vi "32路模拟量输入.vi"() -> ()   [LabVIEW 2010]
uses:
  全局量/全局_配置.vi
panel:
  in  "同步_1":i32
  in  "数组_反馈值":dbl[][](array[numeric])
  in  "第几个数据":i32
  in  "第几组数据":i32
  out "数组_AD幅值":sgl[](array[numeric])
  out "数组_DSP幅值":sgl[](array[numeric])
  in  "数组_设定值":dbl[][](array[numeric])
  in  "数组_选择":bool[](array[boolean])
  out "light_32":bool
  out "light_31":bool
  out "light_30":bool
  out "light_29":bool
  out "light_28":bool
  out "light_27":bool
  out "light_26":bool
  out "light_25":bool
  out "light_24":bool
  out "light_23":bool
  out "light_22":bool
  out "light_21":bool
  out "light_20":bool
  out "light_19":bool
  out "light_18":bool
  out "light_17":bool
  out "Analog_back":string[][](table) caption="表格"
  in  "A_32":bool
  in  "A_31":bool
  in  "A_30":bool
  in  "A_29":bool
  in  "A_28":bool
  in  "A_27":bool
  in  "A_26":bool
  in  "A_25":bool
  in  "A_24":bool
  in  "A_23":bool
  in  "A_22":bool
  in  "A_21":bool
  in  "A_20":bool
  in  "A_19":bool
  in  "A_18":bool
  in  "A_17":bool
  out "合格？":bool[][](array[boolean])
  out "测试结论":string
  out "light_16":bool
  out "light_15":bool
  out "light_14":bool
  out "light_13":bool
  out "light_12":bool
  out "light_11":bool
  out "light_10":bool
  out "light_9":bool
  out "light_8":bool
  out "light_7":bool
  out "light_6":bool
  out "light_5":bool
  out "light_4":bool
  out "light_3":bool
  out "light_2":bool
  out "light_1":bool
  out "退出？":bool
  in  "btn_反选":bool
  in  "btn_全选":bool
  in  "A_16":bool
  in  "A_15":bool
  in  "A_14":bool
  in  "A_13":bool
  in  "A_12":bool
  in  "A_11":bool
  in  "A_10":bool
  in  "A_9":bool
  in  "A_8":bool
  in  "A_7":bool
  in  "A_6":bool
  in  "A_5":bool
  in  "A_4":bool
  in  "A_3":bool
  in  "A_2":bool
  in  "A_1":bool
  in  "btn_取消":bool
  in  "btn_开始测试":bool
  in  "Analog_IN":string[][](table) caption="表格"
  out "Analog_WC":string[][](table) caption="表格"
  # "模拟量选择及输入值（V）"
  # "模拟量反馈值（V）"
  # "模拟量误差值（%）"
  # "测试结论："
  # "从0开始"
  # "从1开始,第0列没有使用"
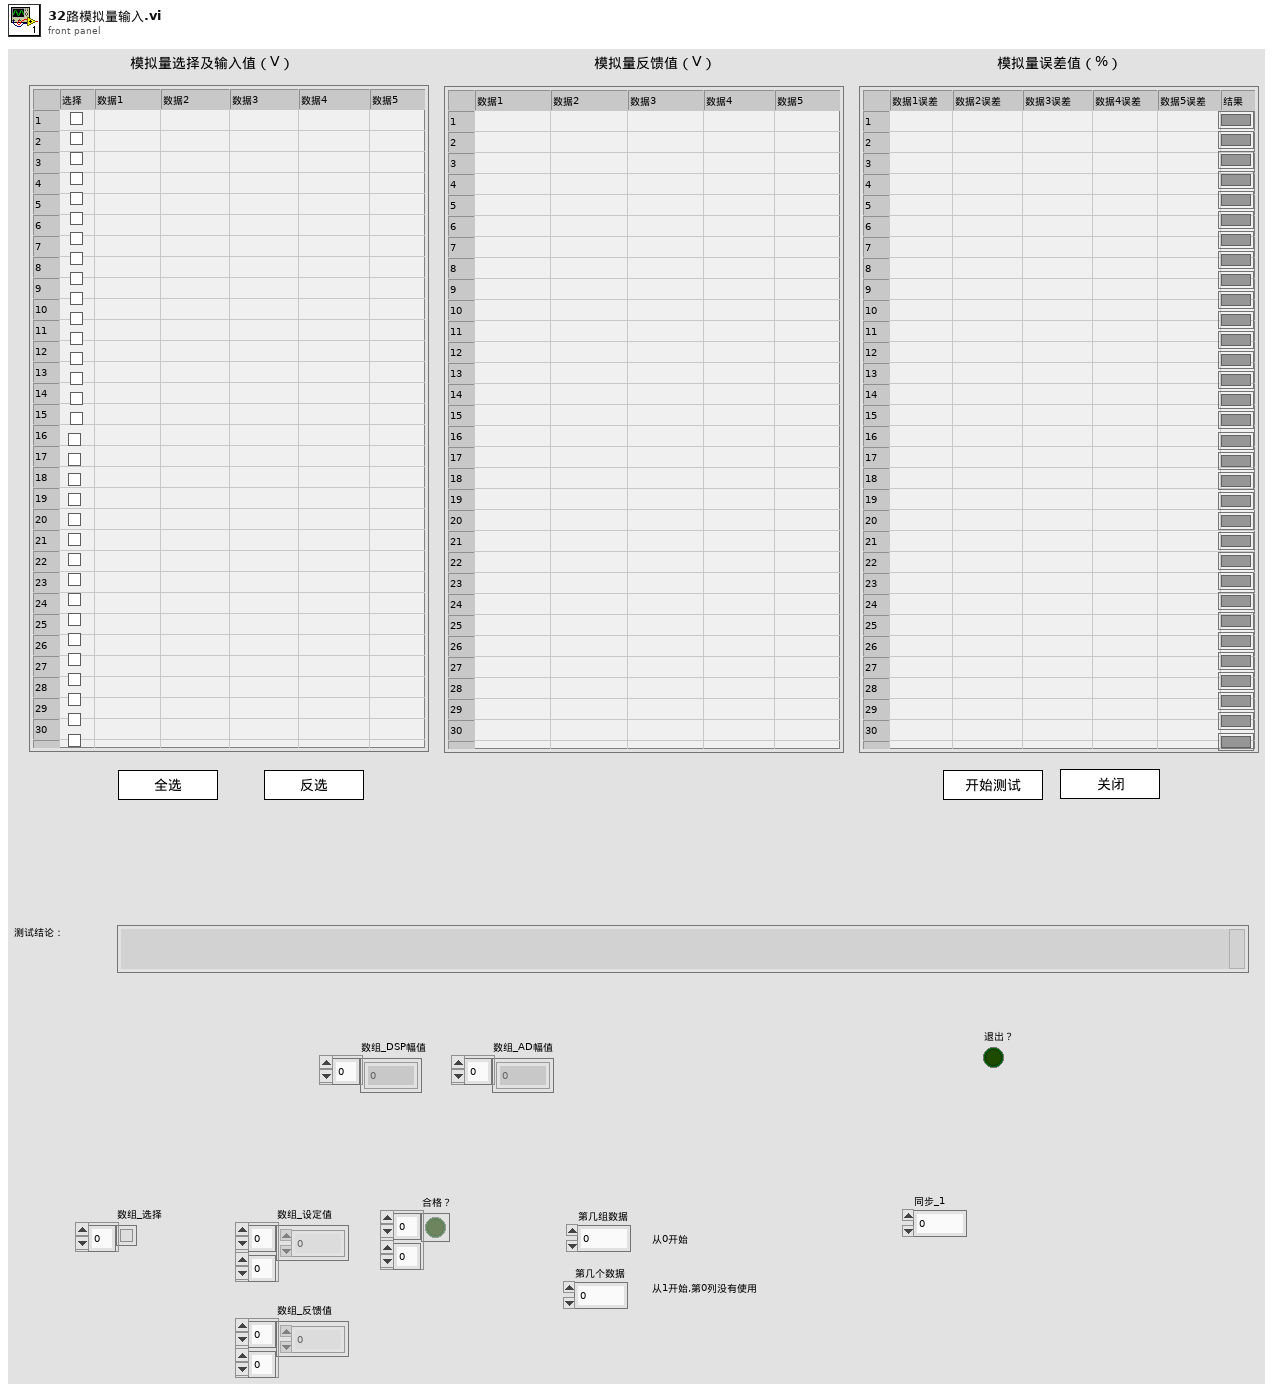
[diagram p1: front panel]
types:
  T1 = enum8{"Enabled", "Disabled", "Disabled and Grayed Out"}
  T2 = cluster{"数字量输入信号路数":u32, "数字量输出信号路数":u32, "DSP模拟量输入信号路数":u32, "DSP模拟量输入信号幅值":u32, "AD模拟量输入信号路数":u32, "AD模拟量输入信号幅值":u32, "RS232端口":u32, "RS232通信路数":u32, "RS232波特率":u32, "RS485端口":u32, "RS485通信路数":u32, "RS485波特率":u32, "CAN通信端口":string, "CAN波特率":u32, "以太网选择?":bool, "控制板IP":string, "以太网端口":u32}
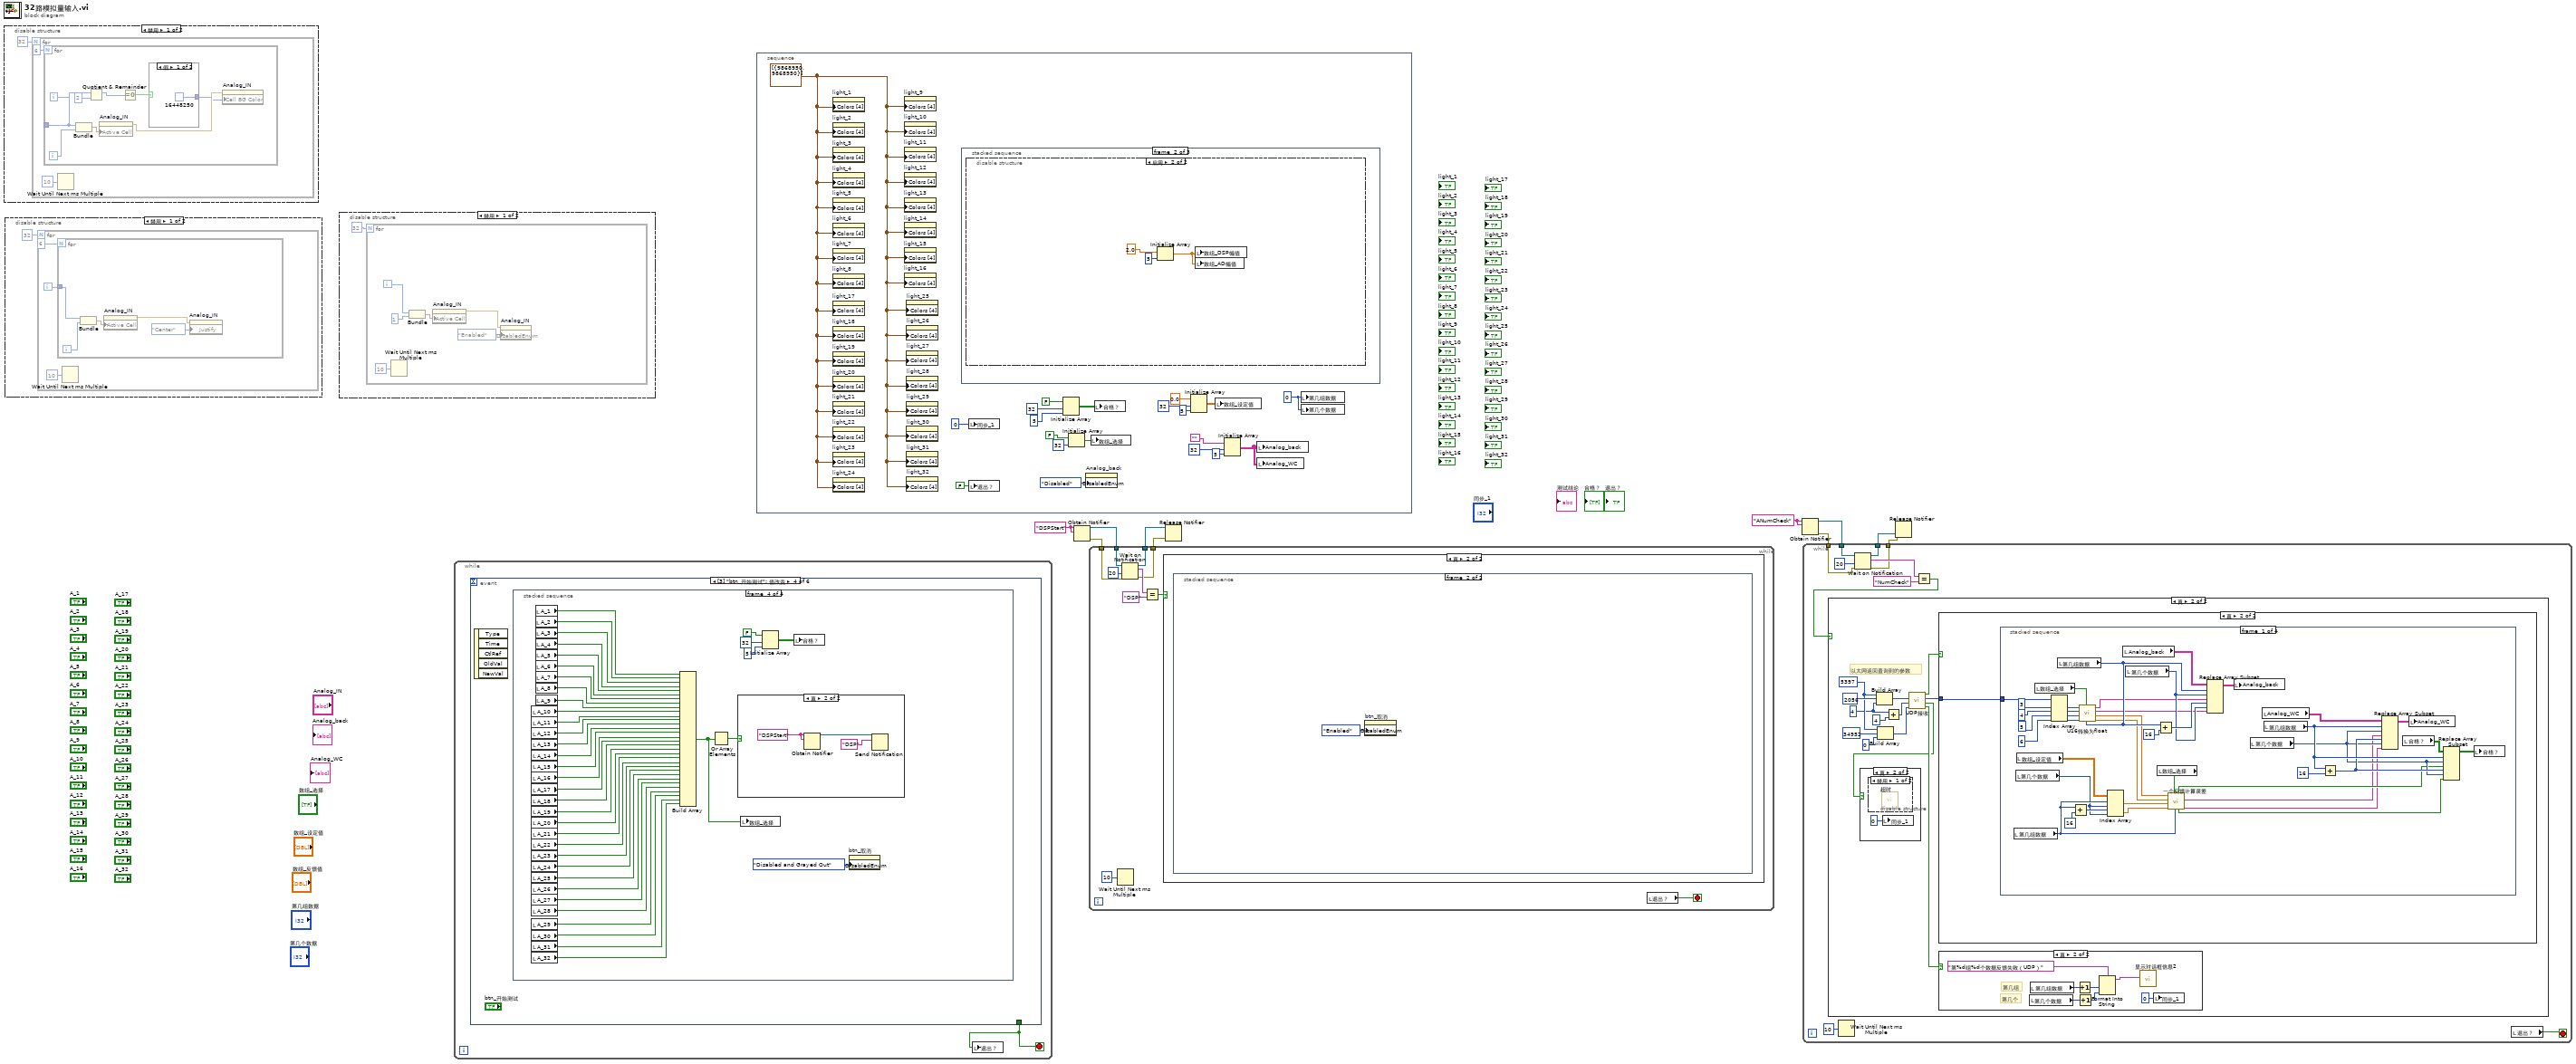
[diagram p0: block diagram]
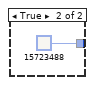
[diagram p2: hidden frame]
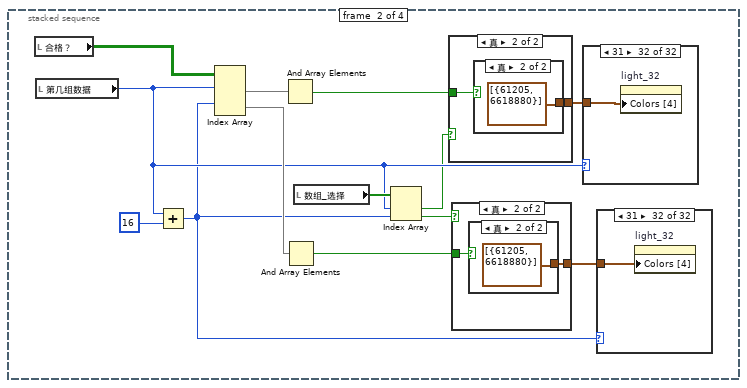
[diagram p9: hidden frame]
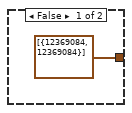
[diagram p10: hidden frame]
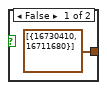
[diagram p11: hidden frame]
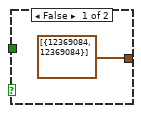
[diagram p12: hidden frame]
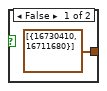
[diagram p13: hidden frame]
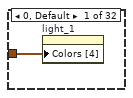
[diagram p14: hidden frame]
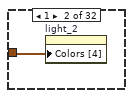
[diagram p15: hidden frame]
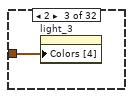
[diagram p16: hidden frame]
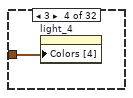
[diagram p17: hidden frame]
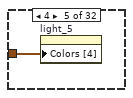
[diagram p18: hidden frame]
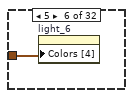
[diagram p19: hidden frame]
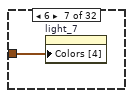
[diagram p20: hidden frame]
diagram:
  w5 = "ANumCheck" ("名称（未命名）")
  w8 = "DSPStart" ("名称（未命名）")
  n1 = disable-structure shown="禁用" {
    frame Disabled {
      n2 = for {
        N: 32 -> [_]
        i -> [w13]
        n3 = for {
          N: 6 -> [_]
          tunnel: w13 -> [w21]
          i -> [w15]
          n4 = Bundle(w21, w15) -> (w18:cluster{i32, i32})  [unwired: 1 in]
          n5 = Quotient & Remainder(x=w21, y=2) -> (x-y*floor(x/y)=w19:i32)  [unwired: 1 out]
          n6 = property on="Analog_IN" class="Tbl (严格)"("Active Cell"=w18) -> (error out=w17:errorcluster)  [unwired: 2 in, 1 out]
          n7 = Equal To 0?(x=w19) -> (x = 0?=w22:bool)
          n8 = case shown="假" w22 {
            tunnel: [u32 16448250 u32 15723488] -> w16
            frame False {
            }
            frame True {
            }
          }
          n9 = property on="Analog_IN" class="Tbl (严格)"(error in=w17, "Cell BG Color"=w16) -> ()  [unwired: 1 in, 2 out]
        }
        n10 = Wait Until Next ms Multiple(millisecond multiple=u32 10 ("毫秒倍数")) -> ()  [unwired: 1 out]
      }
    }
    frame Enabled {
    }
  }
  n11 = disable-structure shown="禁用" {
    frame Disabled {
      n12 = for {
        N: 32 -> [_]
        i -> [w26]
        n13 = for {
          N: 6 -> [_]
          tunnel: w26 -> [w29]
          i -> [w30]
          n14 = Bundle(w29, w30) -> (w33:cluster{i32, i32})  [unwired: 1 in]
          n15 = property on="Analog_IN" class="Tbl (严格)"("Active Cell"=w33) -> (error out=w31:errorcluster)  [unwired: 2 in, 1 out]
          n16 = property on="Analog_IN" class="Tbl (严格)"(error in=w31, "Justify"=enum16{"Left", "Center", "Right"}."Center" ("活动单元格:单元格对齐")) -> ()  [unwired: 1 in, 2 out]
        }
        n17 = Wait Until Next ms Multiple(millisecond multiple=u32 10 ("毫秒倍数")) -> ()  [unwired: 1 out]
      }
    }
    frame Enabled {
    }
  }
  n18 = disable-structure shown="禁用" {
    frame Disabled {
      n19 = for {
        N: 32 -> [_]
        i -> [w39]
        n20 = Wait Until Next ms Multiple(millisecond multiple=u32 10 ("毫秒倍数")) -> ()  [unwired: 1 out]
        n21 = Bundle(w39, 1) -> (w38:cluster{i32, i32})  [unwired: 1 in]
        n22 = property on="Analog_IN" class="Tbl (严格)"("Active Cell"=w38) -> (error out=w35:errorcluster)  [unwired: 2 in, 1 out]
        n23 = property on="Analog_IN" class="Tbl (严格)"(error in=w35, "DisabledEnum"=T1."Enabled" ("禁用")) -> ()  [unwired: 1 in, 2 out]
      }
    }
    frame Enabled {
    }
  }
  n24 = while {
    stop <- w41 stop-if-true
    n25 = event shown="[3] \"btn_开始测试\": 值改变" {
      selector: _ -> [_ _ _ _ _ _]
      dyn-events: _ -> [_ _ _ _ _ _]
      timeout: _ -> [_ _ _ _ _ _]
      tunnel: [_ TRUE TRUE _ _ _] -> w41
      event Timeout {
        n26 = event-data() -> ()  [unwired: 1 in, 2 out]
      }
      event Panel Close {
        n27 = event-data() -> ()  [unwired: 1 in, 3 out]
      }
      event "btn_取消": Value Change {
        n28 = event-data() -> ()  [unwired: 1 in, 5 out]
      }
      event "btn_开始测试": Value Change {
        n29 = event-data() -> ()  [unwired: 1 in, 5 out]
        n30 = stacked-sequence {
          frame #0 {
            w44 = 0 ("第几组数据")
            n31 = local read "Analog_IN"() -> (w51:string[][])
            n32 = Delete From Array(array=w51, length=1 ("长度"), index (col)=0 ("禁用的索引 (列)")) -> (array with subset deleted=w47:string[][])  [unwired: 1 in, 1 out]
            n33 = for {
              N: 32 -> [_]
              tunnel: w47 -> [w54] mode=indexing
              tunnel: [w53] -> w50 mode=indexing
              n34 = for {
                N: 5 -> [_]
                tunnel: w54 -> [w56] mode=indexing
                tunnel: [w55] -> w53 mode=indexing
                n35 = Fract/Exp String To Number(string=w56) -> (number=w55:dbl)  [unwired: 3 in, 1 out]
              }
            }
            n36 = local write "第几组数据"(w44) -> ()
            n37 = local write "第几个数据"(w44) -> ()
            n38 = local write "同步_1"(0 ("同步_2")) -> ()
            n39 = local write "数组_设定值"(w50) -> ()
          }
          frame #1 {
            n40 = local read "Analog_back"() -> (w59:string[][])
            n41 = local read "Analog_WC"() -> (w58:string[][])
            n42 = for {
              tunnel: w58 -> [w95] mode=indexing
              i -> [w94]
              n43 = for {
                tunnel: w95 -> [_] mode=indexing
                tunnel: w94 -> [w99]
                i -> [w98]
                n44 = local read "Analog_WC"() -> (w100:string[][])
                n45 = Replace Array Subset(array=w100, new element="", index (row)=w99, index (col)=w98) -> (w96:string[][])
                n46 = local write "Analog_WC"(w96) -> ()
              }
            }
            n47 = for {
              tunnel: w59 -> [w102] mode=indexing
              i -> [w101]
              n48 = for {
                tunnel: w102 -> [_] mode=indexing
                tunnel: w101 -> [w106]
                i -> [w105]
                n49 = local read "Analog_back"() -> (w107:string[][])
                n50 = Replace Array Subset(array=w107, new element="", index (row)=w106, index (col)=w105) -> (w103:string[][])
                n51 = local write "Analog_back"(w103) -> ()
              }
            }
            n52 = for {
              N: 32 -> [_]
              i -> [w61]
              n53 = case shown="31" w61 {
                tunnel: cluster{u32, u32}[] [{9868950, 9868950}] -> [w62 w63 w64 w65 w66 w67 w68 w69 w70 w71 w72 w73 w74 w75 w76 w77 w78 w79 w80 w81 w82 w83 w84 w85 w86 w87 w88 w89 w90 w91 w92 w93]
                frame 0, Default {
                  n54 = property on="light_1" class="Bool (严格)"("Colors [4]"=w62) -> ()  [unwired: 2 in, 2 out]
                }
                frame 1 {
                  n55 = property on="light_2" class="Bool (严格)"("Colors [4]"=w63) -> ()  [unwired: 2 in, 2 out]
                }
                frame 2 {
                  n56 = property on="light_3" class="Bool (严格)"("Colors [4]"=w64) -> ()  [unwired: 2 in, 2 out]
                }
                frame 3 {
                  n57 = property on="light_4" class="Bool (严格)"("Colors [4]"=w65) -> ()  [unwired: 2 in, 2 out]
                }
                frame 4 {
                  n58 = property on="light_5" class="Bool (严格)"("Colors [4]"=w66) -> ()  [unwired: 2 in, 2 out]
                }
                frame 5 {
                  n59 = property on="light_6" class="Bool (严格)"("Colors [4]"=w67) -> ()  [unwired: 2 in, 2 out]
                }
                frame 6 {
                  n60 = property on="light_7" class="Bool (严格)"("Colors [4]"=w68) -> ()  [unwired: 2 in, 2 out]
                }
                frame 7 {
                  n61 = property on="light_8" class="Bool (严格)"("Colors [4]"=w69) -> ()  [unwired: 2 in, 2 out]
                }
                frame 8 {
                  n62 = property on="light_9" class="Bool (严格)"("Colors [4]"=w70) -> ()  [unwired: 2 in, 2 out]
                }
                frame 9 {
                  n63 = property on="light_10" class="Bool (严格)"("Colors [4]"=w71) -> ()  [unwired: 2 in, 2 out]
                }
                frame 10 {
                  n64 = property on="light_11" class="Bool (严格)"("Colors [4]"=w72) -> ()  [unwired: 2 in, 2 out]
                }
                frame 11 {
                  n65 = property on="light_12" class="Bool (严格)"("Colors [4]"=w73) -> ()  [unwired: 2 in, 2 out]
                }
                frame 12 {
                  n66 = property on="light_13" class="Bool (严格)"("Colors [4]"=w74) -> ()  [unwired: 2 in, 2 out]
                }
                frame 13 {
                  n67 = property on="light_14" class="Bool (严格)"("Colors [4]"=w75) -> ()  [unwired: 2 in, 2 out]
                }
                frame 14 {
                  n68 = property on="light_15" class="Bool (严格)"("Colors [4]"=w76) -> ()  [unwired: 2 in, 2 out]
                }
                frame 15 {
                  n69 = property on="light_16" class="Bool (严格)"("Colors [4]"=w77) -> ()  [unwired: 2 in, 2 out]
                }
                frame 16 {
                  n70 = property on="light_17" class="Bool (严格)"("Colors [4]"=w78) -> ()  [unwired: 2 in, 2 out]
                }
                frame 17 {
                  n71 = property on="light_18" class="Bool (严格)"("Colors [4]"=w79) -> ()  [unwired: 2 in, 2 out]
                }
                frame 18 {
                  n72 = property on="light_19" class="Bool (严格)"("Colors [4]"=w80) -> ()  [unwired: 2 in, 2 out]
                }
                frame 19 {
                  n73 = property on="light_20" class="Bool (严格)"("Colors [4]"=w81) -> ()  [unwired: 2 in, 2 out]
                }
                frame 20 {
                  n74 = property on="light_21" class="Bool (严格)"("Colors [4]"=w82) -> ()  [unwired: 2 in, 2 out]
                }
                frame 21 {
                  n75 = property on="light_22" class="Bool (严格)"("Colors [4]"=w83) -> ()  [unwired: 2 in, 2 out]
                }
                frame 22 {
                  n76 = property on="light_23" class="Bool (严格)"("Colors [4]"=w84) -> ()  [unwired: 2 in, 2 out]
                }
                frame 23 {
                  n77 = property on="light_24" class="Bool (严格)"("Colors [4]"=w85) -> ()  [unwired: 2 in, 2 out]
                }
                frame 24 {
                  n78 = property on="light_25" class="Bool (严格)"("Colors [4]"=w86) -> ()  [unwired: 2 in, 2 out]
                }
                frame 25 {
                  n79 = property on="light_26" class="Bool (严格)"("Colors [4]"=w87) -> ()  [unwired: 2 in, 2 out]
                }
                frame 26 {
                  n80 = property on="light_27" class="Bool (严格)"("Colors [4]"=w88) -> ()  [unwired: 2 in, 2 out]
                }
                frame 27 {
                  n81 = property on="light_28" class="Bool (严格)"("Colors [4]"=w89) -> ()  [unwired: 2 in, 2 out]
                }
                frame 28 {
                  n82 = property on="light_29" class="Bool (严格)"("Colors [4]"=w90) -> ()  [unwired: 2 in, 2 out]
                }
                frame 29 {
                  n83 = property on="light_30" class="Bool (严格)"("Colors [4]"=w91) -> ()  [unwired: 2 in, 2 out]
                }
                frame 30 {
                  n84 = property on="light_31" class="Bool (严格)"("Colors [4]"=w92) -> ()  [unwired: 2 in, 2 out]
                }
                frame 31 {
                  n85 = property on="light_32" class="Bool (严格)"("Colors [4]"=w93) -> ()  [unwired: 2 in, 2 out]
                }
              }
            }
          }
          frame #2 {
            n86 = for {
              N: 32 -> [_]
              i -> [w110]
              n87 = disable-structure shown="禁用" {
                frame Disabled {
                  n88 = Wait Until Next ms Multiple(millisecond multiple=u32 10 ("毫秒倍数")) -> ()  [unwired: 1 out]
                }
                frame Enabled {
                }
              }
              n89 = for {
                N: 6 -> [_]
                tunnel: w110 -> [w118]
                i -> [w115]
                n90 = Bundle(w118, w115) -> (w114:cluster{i32, i32})  [unwired: 1 in]
                n91 = Quotient & Remainder(x=w118, y=2) -> (x-y*floor(x/y)=w116:i32)  [unwired: 1 out]
                n92 = property on="Analog_WC" class="Tbl (严格)"("Active Cell"=w114) -> (error out=w113:errorcluster)  [unwired: 2 in, 1 out]
                n93 = Equal To 0?(x=w116) -> (x = 0?=w119:bool)
                n94 = case shown="假" w119 {
                  tunnel: [u32 16448250 u32 15723488] -> w112
                  frame False {
                  }
                  frame True {
                  }
                }
                n95 = property on="Analog_WC" class="Tbl (严格)"(error in=w113, "Cell BG Color"=w112) -> ()  [unwired: 1 in, 2 out]
              }
            }
          }
          frame #3 {
            n96 = local read "A_10"() -> (w151:bool)
            n97 = local read "A_11"() -> (w150:bool)
            n98 = local read "A_12"() -> (w149:bool)
            n99 = local read "A_13"() -> (w148:bool)
            n100 = local read "A_14"() -> (w147:bool)
            n101 = local read "A_15"() -> (w146:bool)
            n102 = local read "A_16"() -> (w145:bool)
            n103 = local read "A_17"() -> (w144:bool)
            n104 = local read "A_18"() -> (w143:bool)
            n105 = local read "A_19"() -> (w142:bool)
            n106 = local read "A_20"() -> (w141:bool)
            n107 = local read "A_21"() -> (w140:bool)
            n108 = local read "A_22"() -> (w139:bool)
            n109 = local read "A_23"() -> (w138:bool)
            n110 = local read "A_24"() -> (w137:bool)
            n111 = local read "A_25"() -> (w136:bool)
            n112 = local read "A_26"() -> (w135:bool)
            n113 = local read "A_27"() -> (w134:bool)
            n114 = local read "A_28"() -> (w133:bool)
            n115 = local read "A_29"() -> (w132:bool)
            n116 = local read "A_30"() -> (w131:bool)
            n117 = local read "A_31"() -> (w130:bool)
            n118 = local read "A_32"() -> (w129:bool)
            n119 = local read "A_1"() -> (w160:bool)
            n120 = local read "A_2"() -> (w159:bool)
            n121 = local read "A_3"() -> (w158:bool)
            n122 = local read "A_4"() -> (w157:bool)
            n123 = local read "A_5"() -> (w156:bool)
            n124 = local read "A_6"() -> (w155:bool)
            n125 = local read "A_7"() -> (w154:bool)
            n126 = local read "A_8"() -> (w153:bool)
            n127 = local read "A_9"() -> (w152:bool)
            n128 = Build Array(w160, w159, w158, w157, w156, w155, w154, w153, w152, w151, w150, w149, w148, w147, w146, w145, w144, w143, w142, w141, w140, w139, w138, w137, w136, w135, w134, w133, w132, w131, w130, w129) -> (w123:bool[])
            n129 = Or Array Elements(Boolean array=w123) -> (logical OR=w128:bool)
            n130 = case shown="真" w128 {
              frame False {
                n131 = call "显示对话框信息"() -> ()  [unwired: 10 in, 2 out]
              }
              frame True {
                w162 = "DSPStart" ("名称（未命名）")
                n132 = Obtain Notifier(name (unnamed)=w162, notification data type=w162) -> (notifier out=w161:refnum<notifier>)  [unwired: 2 in, 2 out]
                n133 = Send Notification(notification="DSP" ("通知"), notifier=w161) -> ()  [unwired: 1 in, 2 out]
              }
            }
            n134 = local write "数组_选择"(w123) -> ()
            n135 = Initialize Array(FALSE, 32 ("维数大小"), 5 ("维数大小")) -> (w124:bool[][])
            n136 = local write "合格？"(w124) -> ()
            n137 = property on="btn_取消" class="Bool"("DisabledEnum"=T1."Disabled and Grayed Out" ("禁用")) -> ()  [unwired: 2 in, 2 out]
          }
        }
      }
      event "btn_全选": Value Change {
        w164 = TRUE ("单选_AD_1")
        n138 = event-data() -> ()  [unwired: 1 in, 5 out]
        n139 = local write "A_1"(w164) -> ()
        n140 = local write "A_2"(w164) -> ()
        n141 = local write "A_3"(w164) -> ()
        n142 = local write "A_4"(w164) -> ()
        n143 = local write "A_5"(w164) -> ()
        n144 = local write "A_6"(w164) -> ()
        n145 = local write "A_7"(w164) -> ()
        n146 = local write "A_8"(w164) -> ()
        n147 = local write "A_9"(w164) -> ()
        n148 = local write "A_10"(w164) -> ()
        n149 = local write "A_11"(w164) -> ()
        n150 = local write "A_12"(w164) -> ()
        n151 = local write "A_13"(w164) -> ()
        n152 = local write "A_14"(w164) -> ()
        n153 = local write "A_15"(w164) -> ()
        n154 = local write "A_16"(w164) -> ()
        n155 = local write "A_17"(w164) -> ()
        n156 = local write "A_18"(w164) -> ()
        n157 = local write "A_19"(w164) -> ()
        n158 = local write "A_20"(w164) -> ()
        n159 = local write "A_21"(w164) -> ()
        n160 = local write "A_22"(w164) -> ()
        n161 = local write "A_23"(w164) -> ()
        n162 = local write "A_24"(w164) -> ()
        n163 = local write "A_25"(w164) -> ()
        n164 = local write "A_26"(w164) -> ()
        n165 = local write "A_27"(w164) -> ()
        n166 = local write "A_28"(w164) -> ()
        n167 = local write "A_29"(w164) -> ()
        n168 = local write "A_30"(w164) -> ()
        n169 = local write "A_31"(w164) -> ()
        n170 = local write "A_32"(w164) -> ()
      }
      event "btn_反选": Value Change {
        n171 = event-data() -> ()  [unwired: 1 in, 5 out]
        n172 = local read "A_17"() -> (w196:bool)
        n173 = local read "A_18"() -> (w194:bool)
        n174 = local read "A_19"() -> (w192:bool)
        n175 = local read "A_20"() -> (w190:bool)
        n176 = local read "A_21"() -> (w188:bool)
        n177 = local read "A_22"() -> (w186:bool)
        n178 = local read "A_23"() -> (w184:bool)
        n179 = local read "A_24"() -> (w182:bool)
        n180 = local read "A_25"() -> (w180:bool)
        n181 = local read "A_26"() -> (w178:bool)
        n182 = local read "A_27"() -> (w176:bool)
        n183 = local read "A_28"() -> (w174:bool)
        n184 = local read "A_29"() -> (w172:bool)
        n185 = local read "A_30"() -> (w170:bool)
        n186 = local read "A_31"() -> (w168:bool)
        n187 = local read "A_32"() -> (w166:bool)
        n188 = local read "A_1"() -> (w228:bool)
        n189 = local read "A_2"() -> (w226:bool)
        n190 = local read "A_3"() -> (w225:bool)
        n191 = local read "A_4"() -> (w224:bool)
        n192 = local read "A_5"() -> (w223:bool)
        n193 = local read "A_6"() -> (w222:bool)
        n194 = local read "A_7"() -> (w221:bool)
        n195 = local read "A_8"() -> (w220:bool)
        n196 = local read "A_9"() -> (w219:bool)
        n197 = local read "A_10"() -> (w218:bool)
        n198 = local read "A_11"() -> (w217:bool)
        n199 = local read "A_12"() -> (w216:bool)
        n200 = local read "A_13"() -> (w215:bool)
        n201 = local read "A_14"() -> (w214:bool)
        n202 = local read "A_15"() -> (w213:bool)
        n203 = local read "A_16"() -> (w212:bool)
        n204 = Not(x=w228) -> (.not. x?=w227:bool)
        n205 = Not(x=w226) -> (.not. x?=w197:bool)
        n206 = Not(x=w225) -> (.not. x?=w198:bool)
        n207 = Not(x=w224) -> (.not. x?=w199:bool)
        n208 = Not(x=w223) -> (.not. x?=w200:bool)
        n209 = Not(x=w222) -> (.not. x?=w201:bool)
        n210 = Not(x=w221) -> (.not. x?=w202:bool)
        n211 = Not(x=w220) -> (.not. x?=w203:bool)
        n212 = Not(x=w219) -> (.not. x?=w204:bool)
        n213 = Not(x=w218) -> (.not. x?=w205:bool)
        n214 = Not(x=w217) -> (.not. x?=w206:bool)
        n215 = Not(x=w216) -> (.not. x?=w207:bool)
        n216 = Not(x=w215) -> (.not. x?=w208:bool)
        n217 = Not(x=w214) -> (.not. x?=w209:bool)
        n218 = Not(x=w213) -> (.not. x?=w210:bool)
        n219 = Not(x=w212) -> (.not. x?=w211:bool)
        n220 = Not(x=w196) -> (.not. x?=w195:bool)
        n221 = Not(x=w194) -> (.not. x?=w193:bool)
        n222 = Not(x=w192) -> (.not. x?=w191:bool)
        n223 = Not(x=w190) -> (.not. x?=w189:bool)
        n224 = Not(x=w188) -> (.not. x?=w187:bool)
        n225 = Not(x=w186) -> (.not. x?=w185:bool)
        n226 = Not(x=w184) -> (.not. x?=w183:bool)
        n227 = Not(x=w182) -> (.not. x?=w181:bool)
        n228 = Not(x=w180) -> (.not. x?=w179:bool)
        n229 = Not(x=w178) -> (.not. x?=w177:bool)
        n230 = Not(x=w176) -> (.not. x?=w175:bool)
        n231 = Not(x=w174) -> (.not. x?=w173:bool)
        n232 = Not(x=w172) -> (.not. x?=w171:bool)
        n233 = Not(x=w170) -> (.not. x?=w169:bool)
        n234 = Not(x=w168) -> (.not. x?=w167:bool)
        n235 = Not(x=w166) -> (.not. x?=w165:bool)
        n236 = local write "A_1"(w227) -> ()
        n237 = local write "A_2"(w197) -> ()
        n238 = local write "A_3"(w198) -> ()
        n239 = local write "A_4"(w199) -> ()
        n240 = local write "A_5"(w200) -> ()
        n241 = local write "A_6"(w201) -> ()
        n242 = local write "A_7"(w202) -> ()
        n243 = local write "A_8"(w203) -> ()
        n244 = local write "A_9"(w204) -> ()
        n245 = local write "A_10"(w205) -> ()
        n246 = local write "A_11"(w206) -> ()
        n247 = local write "A_12"(w207) -> ()
        n248 = local write "A_13"(w208) -> ()
        n249 = local write "A_14"(w209) -> ()
        n250 = local write "A_15"(w210) -> ()
        n251 = local write "A_16"(w211) -> ()
        n252 = local write "A_17"(w195) -> ()
        n253 = local write "A_18"(w193) -> ()
        n254 = local write "A_19"(w191) -> ()
        n255 = local write "A_20"(w189) -> ()
        n256 = local write "A_21"(w187) -> ()
        n257 = local write "A_22"(w185) -> ()
        n258 = local write "A_23"(w183) -> ()
        n259 = local write "A_24"(w181) -> ()
        n260 = local write "A_25"(w179) -> ()
        n261 = local write "A_26"(w177) -> ()
        n262 = local write "A_27"(w175) -> ()
        n263 = local write "A_28"(w173) -> ()
        n264 = local write "A_29"(w171) -> ()
        n265 = local write "A_30"(w169) -> ()
        n266 = local write "A_31"(w167) -> ()
        n267 = local write "A_32"(w165) -> ()
      }
    }
    n268 = local write "退出？"(w41) -> ()
  }
  n269 = stacked-sequence {
    frame #0 {
      w229 = 0 ("第几组数据")
      w244 = cluster{u32, u32}[] [{9868950, 9868950}]
      n270 = property on="light_1" class="Bool (严格)"("Colors [4]"=w244) -> ()  [unwired: 2 in, 2 out]
      n271 = property on="light_2" class="Bool (严格)"("Colors [4]"=w244) -> ()  [unwired: 2 in, 2 out]
      n272 = property on="light_3" class="Bool (严格)"("Colors [4]"=w244) -> ()  [unwired: 2 in, 2 out]
      n273 = property on="light_4" class="Bool (严格)"("Colors [4]"=w244) -> ()  [unwired: 2 in, 2 out]
      n274 = property on="light_5" class="Bool (严格)"("Colors [4]"=w244) -> ()  [unwired: 2 in, 2 out]
      n275 = property on="light_6" class="Bool (严格)"("Colors [4]"=w244) -> ()  [unwired: 2 in, 2 out]
      n276 = property on="light_7" class="Bool (严格)"("Colors [4]"=w244) -> ()  [unwired: 2 in, 2 out]
      n277 = property on="light_8" class="Bool (严格)"("Colors [4]"=w244) -> ()  [unwired: 2 in, 2 out]
      n278 = property on="light_17" class="Bool (严格)"("Colors [4]"=w244) -> ()  [unwired: 2 in, 2 out]
      n279 = property on="light_18" class="Bool (严格)"("Colors [4]"=w244) -> ()  [unwired: 2 in, 2 out]
      n280 = property on="light_19" class="Bool (严格)"("Colors [4]"=w244) -> ()  [unwired: 2 in, 2 out]
      n281 = property on="light_20" class="Bool (严格)"("Colors [4]"=w244) -> ()  [unwired: 2 in, 2 out]
      n282 = property on="light_21" class="Bool (严格)"("Colors [4]"=w244) -> ()  [unwired: 2 in, 2 out]
      n283 = property on="light_22" class="Bool (严格)"("Colors [4]"=w244) -> ()  [unwired: 2 in, 2 out]
      n284 = property on="light_23" class="Bool (严格)"("Colors [4]"=w244) -> ()  [unwired: 2 in, 2 out]
      n285 = property on="light_24" class="Bool (严格)"("Colors [4]"=w244) -> ()  [unwired: 2 in, 2 out]
      n286 = property on="light_9" class="Bool (严格)"("Colors [4]"=w244) -> ()  [unwired: 2 in, 2 out]
      n287 = property on="light_10" class="Bool (严格)"("Colors [4]"=w244) -> ()  [unwired: 2 in, 2 out]
      n288 = property on="light_11" class="Bool (严格)"("Colors [4]"=w244) -> ()  [unwired: 2 in, 2 out]
      n289 = property on="light_12" class="Bool (严格)"("Colors [4]"=w244) -> ()  [unwired: 2 in, 2 out]
      n290 = property on="light_13" class="Bool (严格)"("Colors [4]"=w244) -> ()  [unwired: 2 in, 2 out]
      n291 = property on="light_14" class="Bool (严格)"("Colors [4]"=w244) -> ()  [unwired: 2 in, 2 out]
      n292 = property on="light_15" class="Bool (严格)"("Colors [4]"=w244) -> ()  [unwired: 2 in, 2 out]
      n293 = property on="light_16" class="Bool (严格)"("Colors [4]"=w244) -> ()  [unwired: 2 in, 2 out]
      n294 = property on="light_25" class="Bool (严格)"("Colors [4]"=w244) -> ()  [unwired: 2 in, 2 out]
      n295 = property on="light_26" class="Bool (严格)"("Colors [4]"=w244) -> ()  [unwired: 2 in, 2 out]
      n296 = property on="light_27" class="Bool (严格)"("Colors [4]"=w244) -> ()  [unwired: 2 in, 2 out]
      n297 = property on="light_28" class="Bool (严格)"("Colors [4]"=w244) -> ()  [unwired: 2 in, 2 out]
      n298 = property on="light_29" class="Bool (严格)"("Colors [4]"=w244) -> ()  [unwired: 2 in, 2 out]
      n299 = property on="light_30" class="Bool (严格)"("Colors [4]"=w244) -> ()  [unwired: 2 in, 2 out]
      n300 = property on="light_31" class="Bool (严格)"("Colors [4]"=w244) -> ()  [unwired: 2 in, 2 out]
      n301 = property on="light_32" class="Bool (严格)"("Colors [4]"=w244) -> ()  [unwired: 2 in, 2 out]
      n302 = stacked-sequence {
        frame #0 {
          n303 = Initialize Array("", 32 ("维数大小"), 6 ("维数大小")) -> (w249:string[][])
          n304 = local write "Analog_IN"(w249) -> ()
        }
        frame #1 {
          n305 = disable-structure shown="启用" {
            frame Disabled {
              n306 = global read "全局_配置.vi" "BoardConfig"() -> (w257:T2)
              n307 = Unbundle By Name(w257) -> ("DSP模拟量输入信号幅值"=w256:u32, "AD模拟量输入信号幅值"=w255:u32)
              n308 = case shown="2" w255 {
                tunnel: [sgl 3.0 sgl 5.0 sgl 12.0] -> w253
                frame 0, Default {
                }
                frame 1 {
                }
                frame 2 {
                }
              }
              n309 = case shown="0, 默认" w256 {
                tunnel: [sgl 3.0 sgl 5.0 sgl 12.0] -> w254
                frame 0, Default {
                }
                frame 1 {
                }
                frame 2 {
                }
              }
              n310 = for {
                N: 5 -> [_]
                tunnel: w254 -> [w279]
                tunnel: w253 -> [w270]
                tunnel: [w268] -> w259 mode=indexing
                tunnel: [w267] -> w258 mode=indexing
                i -> [w282]
                n311 = Multiply(x=sgl 2.0, y=w279) -> (x*y=w277:sgl)
                n312 = Multiply(x=sgl 2.0, y=w270) -> (x*y=w274:sgl)
                n313 = case shown="4" w282 {
                  tunnel: [sgl 0.05 sgl 0.5 sgl 0.75 sgl 0.95 sgl 0.25] -> w269
                  frame 0, Default {
                  }
                  frame 2 {
                  }
                  frame 3 {
                  }
                  frame 4 {
                  }
                  frame 1 {
                  }
                }
                n314 = Multiply(x=w279, y=sgl -1.0) -> (x*y=w280:sgl)
                n315 = Multiply(x=w270, y=sgl -1.0) -> (x*y=w272:sgl)
                n316 = Multiply(x=w269, y=w277) -> (x*y=w276:sgl)
                n317 = Multiply(x=w269, y=w274) -> (x*y=w275:sgl)
                n318 = Add(x=w276, y=w280) -> (x+y=w268:sgl)
                n319 = Add(x=w275, y=w272) -> (x+y=w267:sgl)
              }
              "数组_DSP幅值" <- w259
              "数组_AD幅值" <- w258
            }
            frame Enabled {
              n320 = Initialize Array(sgl 2.0, 5 ("维数大小")) -> (w290:sgl[])
              n321 = local write "数组_DSP幅值"(w290) -> ()
              n322 = local write "数组_AD幅值"(w290) -> ()
            }
          }
        }
        frame #2 {
          n323 = stacked-sequence {
            frame #0 {
              n324 = for {
                N: 16 -> [_]
                i -> [w292]
                n325 = local read "数组_DSP幅值"() -> (w293:sgl[])
                n326 = for {
                  N: 5 -> [_]
                  tunnel: w293 -> [w300] mode=indexing
                  tunnel: w292 -> [w299]
                  i -> [w297]
                  n327 = local read "Analog_IN"() -> (w303:string[][])
                  n328 = Number To Fractional String(number=w300, precision (6)=i16 2 ("精度(6)")) -> (F-format string=w298:string)  [unwired: 2 in]
                  n329 = Increment(x=w297) -> (x+1=w296:i32)
                  n330 = Replace Array Subset(array=w303, new element=w298, index (row)=w299, index (col)=w296) -> (w302:string[][])
                  n331 = local write "Analog_IN"(w302) -> ()
                  n332 = Wait Until Next ms Multiple(millisecond multiple=u32 2 ("毫秒倍数")) -> ()  [unwired: 1 out]
                }
              }
            }
            frame #1 {
              n333 = for {
                N: 16 -> [_]
                i -> [w306]
                n334 = local read "数组_AD幅值"() -> (w305:sgl[])
                n335 = for {
                  N: 5 -> [_]
                  tunnel: w305 -> [w315] mode=indexing
                  tunnel: w306 -> [w310]
                  i -> [w313]
                  n336 = Add(x=w310, y=16) -> (x+y=w308:i32)
                  n337 = local read "Analog_IN"() -> (w318:string[][])
                  n338 = Number To Fractional String(number=w315, precision (6)=i16 2 ("精度(6)")) -> (F-format string=w314:string)  [unwired: 2 in]
                  n339 = Increment(x=w313) -> (x+1=w312:i32)
                  n340 = Replace Array Subset(array=w318, new element=w314, index (row)=w308, index (col)=w312) -> (w317:string[][])
                  n341 = local write "Analog_IN"(w317) -> ()
                  n342 = Wait Until Next ms Multiple(millisecond multiple=u32 2 ("毫秒倍数")) -> ()  [unwired: 1 out]
                }
              }
            }
          }
        }
      }
      n343 = local write "同步_1"(0 ("同步_2")) -> ()
      n344 = local write "退出？"(FALSE ("退出？")) -> ()
      n345 = Initialize Array(FALSE, 32 ("维数大小"), 5 ("维数大小")) -> (w245:bool[][])
      n346 = Initialize Array(FALSE, 32 ("维数大小")) -> (w233:bool[])
      n347 = property on="Analog_back" class="Tbl (严格)"("DisabledEnum"=T1."Disabled" ("禁用")) -> ()  [unwired: 2 in, 2 out]
      n348 = local write "数组_选择"(w233) -> ()
      n349 = local write "合格？"(w245) -> ()
      n350 = Initialize Array(0.0, 32 ("维数大小"), 5 ("维数大小")) -> (w236:dbl[][])
      n351 = local write "数组_设定值"(w236) -> ()
      n352 = Initialize Array("", 32 ("维数大小"), 5 ("维数大小")) -> (w240:string[][])
      n353 = local write "Analog_back"(w240) -> ()
      n354 = local write "Analog_WC"(w240) -> ()
      n355 = local write "第几组数据"(w229) -> ()
      n356 = local write "第几个数据"(w229) -> ()
    }
  }
  n357 = Obtain Notifier(name (unnamed)=w8, notification data type=w8) -> (notifier out=w10:refnum<notifier>, error out=w9:errorcluster)  [unwired: 2 in, 1 out]
  n358 = while {
    tunnel: w10 -> [w322]
    tunnel: w9 -> [w321]
    tunnel: [w320] -> w7
    tunnel: [w319] -> w6
    stop <- w324 stop-if-true
    n359 = Wait Until Next ms Multiple(millisecond multiple=u32 10 ("毫秒倍数")) -> ()  [unwired: 1 out]
    n360 = Wait on Notification(notifier=w322, timeout in ms (-1)=20 ("超时毫秒(-1)"), error in (no error)=w321) -> (notifier out=w320:refnum<notifier>, notification=w328:string, error out=w319:errorcluster)  [unwired: 1 in, 1 out]
    n361 = Equal?(x=w328, y="DSP" ("通知")) -> (x = y?=w325:bool)
    n362 = case shown="真" w325 {
      frame False {
      }
      frame True {
        n363 = stacked-sequence {
          frame #0 {
            n364 = for {
              N: 16 -> [_]
              i -> [w333]
              n365 = local read "数组_选择"() -> (w336:bool[])
              n366 = disable-structure shown="禁用" {
                frame Disabled {
                  n367 = property on="Analog_IN" class="Tbl (严格)"() -> ("Value"=w338:string[][])  [unwired: 2 in, 2 out]
                  n368 = call "表格至数组.vi"("表格控件"=w338) -> ()  [unwired: 10 in, 1 out]
                }
                frame Enabled {
                }
              }
              n369 = local read "数组_设定值"() -> (w337:dbl[][])
              n370 = Add(x=w333, y=16) -> (x+y=w334:i32)
              n371 = Index Array(array=w336, index #1=w333, index #2=w334) -> (element #1=w331:bool, element #2=w330:bool)
              n372 = Or(x=w331, y=w330) -> (x .or. y?=w335:bool)
              n373 = case shown="真" w335 {
                tunnel: w333 -> [_ w339]
                tunnel: w337 -> [_ w341]
                frame False {
                }
                frame True {
                  n374 = Increment(x=w339) -> (x+1=w342:i32)
                  n375 = To Unsigned Byte Integer(number=w342) -> (unsigned 8bit integer=w343:u8)
                  n376 = call "一组模拟量CAN切换开关.vi"("第几组数据"=w343) -> ()  [unwired: 10 in, 1 out]
                  n377 = case shown="真" TRUE {
                    tunnel: w339 -> [_ w344]
                    tunnel: w341 -> [_ w345]
                    frame False {
                    }
                    frame True {
                      n378 = local write "第几组数据"(w344) -> ()
                      n379 = for {
                        N: 5 -> [_]
                        tunnel: w344 -> [w349]
                        tunnel: w345 -> [w348]
                        i -> [w347]
                        n380 = while {
                          tunnel: w349 -> [w357]
                          tunnel: w348 -> [w356]
                          tunnel: w347 -> [w355]
                          stop <- w352 stop-if-true
                          n381 = local read "同步_1"() -> (w353:i32)
                          n382 = Wait Until Next ms Multiple(millisecond multiple=u32 10 ("毫秒倍数")) -> ()  [unwired: 1 out]
                          n383 = Equal?(x=w353, y=0) -> (x = y?=w354:bool)
                          n384 = case shown="真" w354 {
                            tunnel: w357 -> [_ w362]
                            tunnel: w356 -> [_ w361]
                            tunnel: w355 -> [_ w360]
                            tunnel: [FALSE w359] -> w352
                            frame False {
                            }
                            frame True {
                              n385 = stacked-sequence {
                                tunnel: w362 -> [_ w368 _ _ w386 _]
                                tunnel: w361 -> [_ w371 _ _ _ _]
                                tunnel: w360 -> [_ w364 _ _ _ _]
                                tunnel: [_ _ _ _ _ w387] -> w359
                                frame #0 {
                                n386 = Wait (ms)(milliseconds to wait=u32 100) -> ()  [unwired: 1 out]
                                }
                                frame #1 {
                                # "PCI板卡下发模拟量数据"
                                n387 = To Long Integer(number=w368) -> (32bit integer=w367:i32)
                                n388 = local write "第几个数据"(w364) -> ()
                                n389 = Add(x=w367, y=16) -> (x+y=w369:i32)
                                n390 = Index Array(array=w371, index (row) #1=w367, index (col) #1=w364, index (row) #2=w369, index (col) #2=w364) -> (element #1=w366:dbl, element #2=w365:dbl)
                                n391 = Build Array(w366, w365) -> (w372:dbl[])
                                n392 = call "Convert to Dynamic Data"("Array"=w372) -> ("Dynamic Data Type"=w373:dynamicdata)  [unwired: 3 out]
                                n393 = call "DAQNavi Assistant"("data in(DDT)"=w373) -> ()  [unwired: 2 in, 17 out]
                                }
                                frame #2 {
                                w376 = "ANumCheck" ("名称（未命名）")
                                n394 = Obtain Notifier(name (unnamed)=w376, notification data type=w376) -> (notifier out=w375:refnum<notifier>)  [unwired: 2 in, 2 out]
                                n395 = local write "同步_1"(1 ("同步_1")) -> ()
                                n396 = Send Notification(notification="NumCheck" ("通知"), notifier=w375) -> ()  [unwired: 1 in, 2 out]
                                }
                                frame #3 {
                                n397 = Wait (ms)(milliseconds to wait=u32 150) -> ()  [unwired: 1 out]
                                }
                                frame #4 {
                                # "待定"
                                # "待定"
                                # "待定"
                                # "以太网发送读取参数命令"
                                n398 = To Unsigned Word Integer(number=w386) -> (unsigned 16bit integer=w382:u16)
                                n399 = Add(x=w382, y=u16 16) -> (x+y=w383:u16)
                                n400 = Build Array(w382, w383) -> (w385:u16[])
                                n401 = call "UDP发送.vi"("发送数据"=w385, "数据区字长"=u16 2, "报文类型"=u16 2056, "发送方标识"=u16 5397) -> ()  [unwired: 6 in, 1 out]
                                }
                                frame #5 {
                                n402 = local read "同步_1"() -> (w389:i32)
                                n403 = Equal?(x=w389, y=1) -> (x = y?=w387:bool)
                                }
                              }
                            }
                          }
                        }
                      }
                    }
                  }
                }
              }
            }
          }
          frame #1 {
            n404 = property on="btn_取消" class="Bool"("DisabledEnum"=T1."Enabled" ("禁用")) -> ()  [unwired: 2 in, 2 out]
          }
        }
      }
    }
    n405 = local read "退出？"() -> (w324:bool)
  }
  n406 = Release Notifier(notifier=w7, error in (no error)=w6) -> ()  [unwired: 1 in, 3 out]
  n407 = Obtain Notifier(name (unnamed)=w5, notification data type=w5) -> (notifier out=w4:refnum<notifier>, error out=w3:errorcluster)  [unwired: 2 in, 1 out]
  n408 = while {
    tunnel: w4 -> [w395]
    tunnel: w3 -> [w394]
    tunnel: [w393] -> w2
    tunnel: [w392] -> w1
    stop <- w391 stop-if-true
    n409 = Wait Until Next ms Multiple(millisecond multiple=u32 10 ("毫秒倍数")) -> ()  [unwired: 1 out]
    n410 = Wait on Notification(notifier=w395, timeout in ms (-1)=20 ("超时毫秒(-1)"), error in (no error)=w394) -> (notifier out=w393:refnum<notifier>, notification=w398:string, error out=w392:errorcluster)  [unwired: 1 in, 1 out]
    n411 = Equal?(x=w398, y="NumCheck" ("通知")) -> (x = y?=w396:bool)
    n412 = case shown="真" w396 {
      frame False {
      }
      frame True {
        w403 = u16 4
        w412 = u16 5397
        # "以太网返回查询到的参数"
        n413 = Build Array(w412, u16 2056, w403) -> (w409:u16[])
        n414 = Build Array(w412, u16 34952, u16 0 ("元素")) -> (w408:u16[])
        n415 = Add(x=w403, y=u16 4) -> (x+y=w401:u16)
        n416 = call "UDP接收.vi"("匹配帧信息_异常"=w408, "长度"=w401, "匹配帧信息_正常"=w409) -> ("异常_找到?"=w405:bool, "接收超时?"=w404:bool, "接收的一帧数据"=w406:u16[], "正常_找到?"=w407:bool)  [unwired: 5 in]
        n417 = case shown="真" w404 {
          frame False {
          }
          frame True {
            n418 = disable-structure shown="禁用" {
              frame Disabled {
                n419 = call "超时"() -> ()  [unwired: 10 in, 2 out]
              }
              frame Enabled {
              }
            }
            n420 = local write "同步_1"(0 ("同步_1")) -> ()
          }
        }
        n421 = case shown="真" w407 {
          tunnel: w406 -> [_ w422]
          frame False {
          }
          frame True {
            n422 = stacked-sequence {
              tunnel: w422 -> [w462 _ _ _]
              frame #0 {
                n423 = local read "第几组数据"() -> (w430:i32)
                n424 = local read "第几个数据"() -> (w425:i32)
                n425 = local read "数组_设定值"() -> (w456:dbl[][])
                n426 = local read "数组_选择"() -> (w434:bool[])
                n427 = Index Array(array=w462, index #1=3 ("索引"), index #2=4 ("索引"), index #3=5 ("索引"), index #4=6 ("索引")) -> (element #1=w441:u16, element #2=w440:u16, element #3=w439:u16, element #4=w438:u16)
                n428 = local read "第几组数据"() -> (w437:i32)
                n429 = Add(x=w430, y=16) -> (x+y=w443:i32)
                n430 = call "U16转换为float.vi"("第几组数据"=w437, "选择?"=w434, "低16位_2"=w438, "高16位_2"=w439, "低16位_1"=w440, "高16位_1"=w441) -> ("反馈值2"=w432:dbl, "反馈值1"=w423:dbl, "反馈值字符_2"=w435:string, "反馈值字符_1"=w436:string)  [unwired: 2 in]
                n431 = Index Array(array=w456, index (row) #1=w430, index (col) #1=w425, index (row) #2=w443, index (col) #2=w425) -> (element #1=w424:dbl, element #2=w431:dbl)
                n432 = local read "Analog_back"() -> (w448:string[][])
                n433 = local read "第几个数据"() -> (w442:i32)
                n434 = local read "数组_选择"() -> (w433:bool[])
                n435 = Add(x=w437, y=16) -> (x+y=w446:i32)
                n436 = call "一个反馈计算误差.vi"("第几组"=w430, "选择?"=w433, "设定值_2"=w431, "设定值_1"=w424, "反馈值_2"=w432, "反馈值_1"=w423) -> ("字符串_误差_2"=w427:string, "字符串_误差_1"=w428:string, "合格_2?"=w426:bool, "合格_1?"=w429:bool)  [unwired: 2 out]
                n437 = Replace Array Subset(array=w448, new element #1=w436, index (row) #1=w437, index (col) #1=w442, new element #2=w435, index (row) #2=w446, index (col) #2=w442) -> (w447:string[][])
                n438 = local write "Analog_back"(w447) -> ()
                n439 = local read "第几个数据"() -> (w444:i32)
                n440 = local read "Analog_WC"() -> (w453:string[][])
                n441 = local read "第几组数据"() -> (w451:i32)
                n442 = Add(x=w451, y=16) -> (x+y=w445:i32)
                n443 = Replace Array Subset(array=w453, new element #1=w428, index (row) #1=w451, index (col) #1=w444, new element #2=w427, index (row) #2=w445, index (col) #2=w444) -> (w452:string[][])
                n444 = local read "合格？"() -> (w449:bool[][])
                n445 = local write "Analog_WC"(w452) -> ()
                n446 = Replace Array Subset(array=w449, new element #1=w429, index (row) #1=w451, index (col) #1=w444, new element #2=w426, index (row) #2=w445, index (col) #2=w444) -> (w450:bool[][])
                n447 = local write "合格？"(w450) -> ()
              }
              frame #1 {
                n448 = local read "合格？"() -> (w472:bool[][])
                n449 = local read "第几组数据"() -> (w466:i32)
                n450 = Add(x=w466, y=16) -> (x+y=w465:i32)
                n451 = Index Array(array=w472, index (row) #1=w466, index (row) #2=w465) -> (element #1=w475:bool[], element #2=w469:bool[])  [unwired: 2 in]
                n452 = And Array Elements(Boolean array=w475) -> (logical AND=w470:bool)
                n453 = And Array Elements(Boolean array=w469) -> (logical AND=w468:bool)
                n454 = local read "数组_选择"() -> (w467:bool[])
                n455 = Index Array(array=w467, index #1=w466, index #2=w465) -> (element #1=w464:bool, element #2=w463:bool)
                n456 = case shown="真" w464 {
                  tunnel: [cluster{u32, u32}[] [{12369084, 12369084}] w483] -> w474
                  tunnel: w470 -> [_ w482]
                  frame False {
                  }
                  frame True {
                    n457 = case shown="真" w482 {
                      tunnel: [cluster{u32, u32}[] [{16730410, 16711680}] cluster{u32, u32}[] [{61205, 6618880}]] -> w483
                      frame False {
                      }
                      frame True {
                      }
                    }
                  }
                }
                n458 = case shown="真" w463 {
                  tunnel: [cluster{u32, u32}[] [{12369084, 12369084}] w478] -> w471
                  tunnel: w468 -> [_ w477]
                  frame False {
                  }
                  frame True {
                    n459 = case shown="真" w477 {
                      tunnel: [cluster{u32, u32}[] [{16730410, 16711680}] cluster{u32, u32}[] [{61205, 6618880}]] -> w478
                      frame False {
                      }
                      frame True {
                      }
                    }
                  }
                }
                n460 = case shown="31" w466 {
                  tunnel: w474 -> [w518 w519 w520 w521 w522 w523 w524 w525 w526 w527 w528 w529 w530 w531 w532 w533 w534 w535 w536 w537 w538 w539 w540 w541 w542 w543 w544 w545 w546 w547 w548 w549]
                  frame 0, Default {
                    n461 = property on="light_1" class="Bool (严格)"("Colors [4]"=w518) -> ()  [unwired: 2 in, 2 out]
                  }
                  frame 1 {
                    n462 = property on="light_2" class="Bool (严格)"("Colors [4]"=w519) -> ()  [unwired: 2 in, 2 out]
                  }
                  frame 2 {
                    n463 = property on="light_3" class="Bool (严格)"("Colors [4]"=w520) -> ()  [unwired: 2 in, 2 out]
                  }
                  frame 3 {
                    n464 = property on="light_4" class="Bool (严格)"("Colors [4]"=w521) -> ()  [unwired: 2 in, 2 out]
                  }
                  frame 4 {
                    n465 = property on="light_5" class="Bool (严格)"("Colors [4]"=w522) -> ()  [unwired: 2 in, 2 out]
                  }
                  frame 5 {
                    n466 = property on="light_6" class="Bool (严格)"("Colors [4]"=w523) -> ()  [unwired: 2 in, 2 out]
                  }
                  frame 6 {
                    n467 = property on="light_7" class="Bool (严格)"("Colors [4]"=w524) -> ()  [unwired: 2 in, 2 out]
                  }
                  frame 7 {
                    n468 = property on="light_8" class="Bool (严格)"("Colors [4]"=w525) -> ()  [unwired: 2 in, 2 out]
                  }
                  frame 8 {
                    n469 = property on="light_9" class="Bool (严格)"("Colors [4]"=w526) -> ()  [unwired: 2 in, 2 out]
                  }
                  frame 9 {
                    n470 = property on="light_10" class="Bool (严格)"("Colors [4]"=w527) -> ()  [unwired: 2 in, 2 out]
                  }
                  frame 10 {
                    n471 = property on="light_11" class="Bool (严格)"("Colors [4]"=w528) -> ()  [unwired: 2 in, 2 out]
                  }
                  frame 11 {
                    n472 = property on="light_12" class="Bool (严格)"("Colors [4]"=w529) -> ()  [unwired: 2 in, 2 out]
                  }
                  frame 12 {
                    n473 = property on="light_13" class="Bool (严格)"("Colors [4]"=w530) -> ()  [unwired: 2 in, 2 out]
                  }
                  frame 13 {
                    n474 = property on="light_14" class="Bool (严格)"("Colors [4]"=w531) -> ()  [unwired: 2 in, 2 out]
                  }
                  frame 14 {
                    n475 = property on="light_15" class="Bool (严格)"("Colors [4]"=w532) -> ()  [unwired: 2 in, 2 out]
                  }
                  frame 15 {
                    n476 = property on="light_16" class="Bool (严格)"("Colors [4]"=w533) -> ()  [unwired: 2 in, 2 out]
                  }
                  frame 16 {
                    n477 = property on="light_17" class="Bool (严格)"("Colors [4]"=w534) -> ()  [unwired: 2 in, 2 out]
                  }
                  frame 17 {
                    n478 = property on="light_18" class="Bool (严格)"("Colors [4]"=w535) -> ()  [unwired: 2 in, 2 out]
                  }
                  frame 18 {
                    n479 = property on="light_19" class="Bool (严格)"("Colors [4]"=w536) -> ()  [unwired: 2 in, 2 out]
                  }
                  frame 19 {
                    n480 = property on="light_20" class="Bool (严格)"("Colors [4]"=w537) -> ()  [unwired: 2 in, 2 out]
                  }
                  frame 20 {
                    n481 = property on="light_21" class="Bool (严格)"("Colors [4]"=w538) -> ()  [unwired: 2 in, 2 out]
                  }
                  frame 21 {
                    n482 = property on="light_22" class="Bool (严格)"("Colors [4]"=w539) -> ()  [unwired: 2 in, 2 out]
                  }
                  frame 22 {
                    n483 = property on="light_23" class="Bool (严格)"("Colors [4]"=w540) -> ()  [unwired: 2 in, 2 out]
                  }
                  frame 23 {
                    n484 = property on="light_24" class="Bool (严格)"("Colors [4]"=w541) -> ()  [unwired: 2 in, 2 out]
                  }
                  frame 24 {
                    n485 = property on="light_25" class="Bool (严格)"("Colors [4]"=w542) -> ()  [unwired: 2 in, 2 out]
                  }
                  frame 25 {
                    n486 = property on="light_26" class="Bool (严格)"("Colors [4]"=w543) -> ()  [unwired: 2 in, 2 out]
                  }
                  frame 26 {
                    n487 = property on="light_27" class="Bool (严格)"("Colors [4]"=w544) -> ()  [unwired: 2 in, 2 out]
                  }
                  frame 27 {
                    n488 = property on="light_28" class="Bool (严格)"("Colors [4]"=w545) -> ()  [unwired: 2 in, 2 out]
                  }
                  frame 28 {
                    n489 = property on="light_29" class="Bool (严格)"("Colors [4]"=w546) -> ()  [unwired: 2 in, 2 out]
                  }
                  frame 29 {
                    n490 = property on="light_30" class="Bool (严格)"("Colors [4]"=w547) -> ()  [unwired: 2 in, 2 out]
                  }
                  frame 30 {
                    n491 = property on="light_31" class="Bool (严格)"("Colors [4]"=w548) -> ()  [unwired: 2 in, 2 out]
                  }
                  frame 31 {
                    n492 = property on="light_32" class="Bool (严格)"("Colors [4]"=w549) -> ()  [unwired: 2 in, 2 out]
                  }
                }
                n493 = case shown="31" w465 {
                  tunnel: w471 -> [w486 w487 w488 w489 w490 w491 w492 w493 w494 w495 w496 w497 w498 w499 w500 w501 w502 w503 w504 w505 w506 w507 w508 w509 w510 w511 w512 w513 w514 w515 w516 w517]
                  frame 0, Default {
                    n494 = property on="light_1" class="Bool (严格)"("Colors [4]"=w486) -> ()  [unwired: 2 in, 2 out]
                  }
                  frame 1 {
                    n495 = property on="light_2" class="Bool (严格)"("Colors [4]"=w487) -> ()  [unwired: 2 in, 2 out]
                  }
                  frame 2 {
                    n496 = property on="light_3" class="Bool (严格)"("Colors [4]"=w488) -> ()  [unwired: 2 in, 2 out]
                  }
                  frame 3 {
                    n497 = property on="light_4" class="Bool (严格)"("Colors [4]"=w489) -> ()  [unwired: 2 in, 2 out]
                  }
                  frame 4 {
                    n498 = property on="light_5" class="Bool (严格)"("Colors [4]"=w490) -> ()  [unwired: 2 in, 2 out]
                  }
                  frame 5 {
                    n499 = property on="light_6" class="Bool (严格)"("Colors [4]"=w491) -> ()  [unwired: 2 in, 2 out]
                  }
                  frame 6 {
                    n500 = property on="light_7" class="Bool (严格)"("Colors [4]"=w492) -> ()  [unwired: 2 in, 2 out]
                  }
                  frame 7 {
                    n501 = property on="light_8" class="Bool (严格)"("Colors [4]"=w493) -> ()  [unwired: 2 in, 2 out]
                  }
                  frame 8 {
                    n502 = property on="light_9" class="Bool (严格)"("Colors [4]"=w494) -> ()  [unwired: 2 in, 2 out]
                  }
                  frame 9 {
                    n503 = property on="light_10" class="Bool (严格)"("Colors [4]"=w495) -> ()  [unwired: 2 in, 2 out]
                  }
                  frame 10 {
                    n504 = property on="light_11" class="Bool (严格)"("Colors [4]"=w496) -> ()  [unwired: 2 in, 2 out]
                  }
                  frame 11 {
                    n505 = property on="light_12" class="Bool (严格)"("Colors [4]"=w497) -> ()  [unwired: 2 in, 2 out]
                  }
                  frame 12 {
                    n506 = property on="light_13" class="Bool (严格)"("Colors [4]"=w498) -> ()  [unwired: 2 in, 2 out]
                  }
                  frame 13 {
                    n507 = property on="light_14" class="Bool (严格)"("Colors [4]"=w499) -> ()  [unwired: 2 in, 2 out]
                  }
                  frame 14 {
                    n508 = property on="light_15" class="Bool (严格)"("Colors [4]"=w500) -> ()  [unwired: 2 in, 2 out]
                  }
                  frame 15 {
                    n509 = property on="light_16" class="Bool (严格)"("Colors [4]"=w501) -> ()  [unwired: 2 in, 2 out]
                  }
                  frame 16 {
                    n510 = property on="light_17" class="Bool (严格)"("Colors [4]"=w502) -> ()  [unwired: 2 in, 2 out]
                  }
                  frame 17 {
                    n511 = property on="light_18" class="Bool (严格)"("Colors [4]"=w503) -> ()  [unwired: 2 in, 2 out]
                  }
                  frame 18 {
                    n512 = property on="light_19" class="Bool (严格)"("Colors [4]"=w504) -> ()  [unwired: 2 in, 2 out]
                  }
                  frame 19 {
                    n513 = property on="light_20" class="Bool (严格)"("Colors [4]"=w505) -> ()  [unwired: 2 in, 2 out]
                  }
                  frame 20 {
                    n514 = property on="light_21" class="Bool (严格)"("Colors [4]"=w506) -> ()  [unwired: 2 in, 2 out]
                  }
                  frame 21 {
                    n515 = property on="light_22" class="Bool (严格)"("Colors [4]"=w507) -> ()  [unwired: 2 in, 2 out]
                  }
                  frame 22 {
                    n516 = property on="light_23" class="Bool (严格)"("Colors [4]"=w508) -> ()  [unwired: 2 in, 2 out]
                  }
                  frame 23 {
                    n517 = property on="light_24" class="Bool (严格)"("Colors [4]"=w509) -> ()  [unwired: 2 in, 2 out]
                  }
                  frame 24 {
                    n518 = property on="light_25" class="Bool (严格)"("Colors [4]"=w510) -> ()  [unwired: 2 in, 2 out]
                  }
                  frame 25 {
                    n519 = property on="light_26" class="Bool (严格)"("Colors [4]"=w511) -> ()  [unwired: 2 in, 2 out]
                  }
                  frame 26 {
                    n520 = property on="light_27" class="Bool (严格)"("Colors [4]"=w512) -> ()  [unwired: 2 in, 2 out]
                  }
                  frame 27 {
                    n521 = property on="light_28" class="Bool (严格)"("Colors [4]"=w513) -> ()  [unwired: 2 in, 2 out]
                  }
                  frame 28 {
                    n522 = property on="light_29" class="Bool (严格)"("Colors [4]"=w514) -> ()  [unwired: 2 in, 2 out]
                  }
                  frame 29 {
                    n523 = property on="light_30" class="Bool (严格)"("Colors [4]"=w515) -> ()  [unwired: 2 in, 2 out]
                  }
                  frame 30 {
                    n524 = property on="light_31" class="Bool (严格)"("Colors [4]"=w516) -> ()  [unwired: 2 in, 2 out]
                  }
                  frame 31 {
                    n525 = property on="light_32" class="Bool (严格)"("Colors [4]"=w517) -> ()  [unwired: 2 in, 2 out]
                  }
                }
              }
              frame #2 {
                n526 = local read "第几组数据"() -> (w553:i32)
                n527 = Add(x=w553, y=16) -> (x+y=w555:i32)
                n528 = local read "第几个数据"() -> (w557:i32)
                n529 = local read "合格？"() -> (w558:bool[][])
                n530 = local read "数组_选择"() -> (w556:bool[])
                n531 = Index Array(array=w558, index (row) #1=w553, index (col) #1=w557, index (row) #2=w555, index (col) #2=w557) -> (element #1=w554:bool, element #2=w550:bool)
                n532 = Index Array(array=w556, index #1=w553, index #2=w555) -> (element #1=w552:bool, element #2=w551:bool)
                n533 = case shown="真" w552 {
                  tunnel: w557 -> [_ w569]
                  tunnel: w554 -> [_ w568]
                  tunnel: w553 -> [_ w567]
                  frame False {
                  }
                  frame True {
                    n534 = call "误差表格颜色.vi"("合格？"=w568, "第几组"=w567) -> ("颜色"=w566:u32)  [unwired: 9 in]
                    n535 = Bundle("第几组数据"=w567, "第几个数据"=w569) -> (w571:cluster{"第几组数据":i32, "第几个数据":i32})  [unwired: 1 in]
                    n536 = property on="Analog_WC" class="Tbl (严格)"("Active Cell"=w571) -> (error out=w570:errorcluster)  [unwired: 2 in, 1 out]
                    n537 = property on="Analog_WC" class="Tbl (严格)"(error in=w570, "Cell BG Color"=w566) -> ()  [unwired: 1 in, 2 out]
                  }
                }
                n538 = case shown="真" w551 {
                  tunnel: w557 -> [_ w563]
                  tunnel: w555 -> [_ w562]
                  tunnel: w550 -> [_ w560]
                  frame False {
                  }
                  frame True {
                    n539 = Bundle(w562, "第几个数据"=w563) -> (w564:cluster{i32, "第几个数据":i32})  [unwired: 1 in]
                    n540 = call "误差表格颜色.vi"("合格？"=w560, "第几组"=w562) -> ("颜色"=w561:u32)  [unwired: 9 in]
                    n541 = property on="Analog_WC" class="Tbl (严格)"("Active Cell"=w564) -> (error out=w565:errorcluster)  [unwired: 2 in, 1 out]
                    n542 = property on="Analog_WC" class="Tbl (严格)"(error in=w565, "Cell BG Color"=w561) -> ()  [unwired: 1 in, 2 out]
                  }
                }
              }
              frame #3 {
                n543 = flat-sequence {
                  frame #0 {
                    n544 = Wait Until Next ms Multiple(millisecond multiple=u32 100) -> ()  [unwired: 1 out]
                  }
                  frame #1 {
                    n545 = local write "同步_1"(0 ("同步_1")) -> ()
                  }
                }
              }
            }
          }
        }
        n546 = case shown="真" w405 {
          frame False {
          }
          frame True {
            # "第几个"
            # "第几组"
            n547 = local read "第几个数据"() -> (w416:i32)
            n548 = local read "第几组数据"() -> (w418:i32)
            n549 = Increment(x=w418) -> (x+1=w419:i32)
            n550 = Increment(x=w416) -> (x+1=w417:i32)
            n551 = Format Into String(format string="第%d组%d个数据反馈失败（UDP）" ("Message"), w419, w417) -> (resulting string=w420:string)  [unwired: 2 in, 1 out]
            n552 = call "显示对话框信息2"("Message"=w420) -> ()  [unwired: 9 in, 2 out]
            n553 = local write "同步_1"(0 ("同步_1")) -> ()
          }
        }
      }
    }
    n554 = local read "退出？"() -> (w391:bool)
  }
  n555 = Release Notifier(notifier=w2, error in (no error)=w1) -> ()  [unwired: 1 in, 3 out]
